vi "scale.vi"() -> ()   [LabVIEW 2021]
uses:
  <vilib>/DAQmx/read.llb/DAQmx Read (Analog DBL 1Chan 1Samp).vi
  <vilib>/DAQmx/create/channels.llb/DAQmx Create Channel (AI-Voltage-Basic).vi
  <vilib>/DAQmx/configure/timing.llb/DAQmx Timing (Sample Clock).vi
  <vilib>/DAQmx/miscellaneous.llb/DAQmx Fill In Error Info.vi
  <vilib>/DAQmx/create/scale.llb/DAQmx Create Scale (Linear).vi
panel:
  in  "y-intercept":dbl format="%0.2f"
  in  "slope":dbl=1.0 format="%0.2f"
  in  "stop":bool
  out "data":dbl(slide) scale=-5.0..10.0
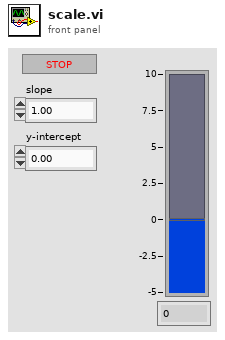
[diagram p1: front panel]
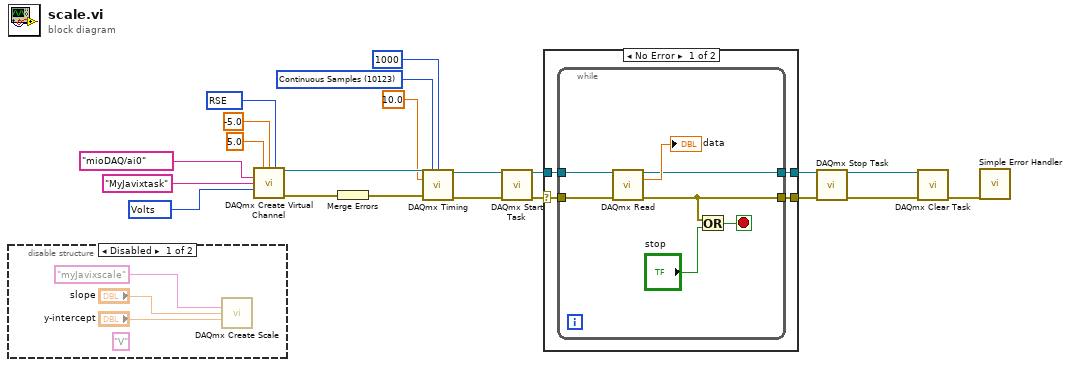
[diagram p0: block diagram]
diagram:
  w4 = 10348 items=["Volts"=10348, "From Custom Scale"=10065] ("units")
  w17 = 10083 items=["Default"=-1, "RSE"=10083, "NRSE"=10078, "Differential"=10106, "Pseudodifferential"=12529] ("input terminal configuration")
  w12 = 10123 items=["Finite Samples"=10178, "Continuous Samples"=10123, "Hardware Timed Single Point"=12522] ("sample mode")
  n1 = disable-structure shown="Disabled" {
    frame Disabled {
      (unwired) "V" ("scaled units")
      n2 = call-poly <vilib>:"DAQmx Create Scale.vi"("name"="myJavixscale", "slope"="slope", "y-intercept"="y-intercept") -> ()  [unwired: 11 in, 2 out]
    }
    frame Enabled {
    }
  }
  n3 = call-poly <vilib>:"DAQmx Create Virtual Channel.vi"("maximum value"=5.0, "minimum value"=-5.0, "input terminal configuration"=w17, "physical channels"=tag "mioDAQ/ai0", "name to assign"="MyJavixtask", "units"=w4) -> ("task out"=w18:refnum<k21>, "error out"=w19:errorcluster)  [unwired: 8 in]
  n4 = Merge Errors(w19) -> (w3:errorcluster)
  n5 = call-poly <vilib>:"DAQmx Timing.vi"("task/channels in"=w18, "sample mode"=w12, "samples per channel"=1000, "rate"=10.0, "error in"=w3) -> ("task out"=w20:refnum<k21>, "error out"=w21:errorcluster)  [unwired: 9 in]
  n6 = call <vilib>:"DAQmx Start Task.vi"("task/channels in"=w20, "error in"=w21) -> ("task out"=w7:refnum<k21>, "error out"=w8:errorcluster)  [unwired: 12 in]
  n7 = case shown="No Error" w8 {
    selector: w8 -> [w28 w36]
    tunnel: w7 -> [w27 w37]
    tunnel: [w26 w37] -> w6
    tunnel: [w25 w36] -> w5
    frame No Error {
      n8 = while {
        tunnel: w28 -> [w34]
        tunnel: w27 -> [w33]
        tunnel: [w32] -> w26
        tunnel: [w31] -> w25
        stop <- w29 stop-if-true
        n9 = call-poly <vilib>:"DAQmx Read.vi"("task/channels in"=w33, "error in"=w34) -> ("task out"=w32:refnum<k21>, "data"=→"data":dbl, "error out"=w31:errorcluster)  [unwired: 11 in]
        n10 = Or(x=w31, y="stop") -> (x .or. y?=w29:bool)
      }
    }
    frame Error {
    }
  }
  n11 = call <vilib>:"DAQmx Stop Task.vi"("task/channels in"=w6, "error in"=w5) -> ("task out"=w10:refnum<k21>, "error out"=w9:errorcluster)  [unwired: 12 in]
  n12 = call <vilib>:"DAQmx Clear Task.vi"("task in"=w10, "error in"=w9) -> ("error out"=w11:errorcluster)  [unwired: 13 in]
  n13 = call <vilib>:"Simple Error Handler.vi"("error in (no error)"=w11) -> ()  [unwired: 4 in, 5 out]
